vi "writeIMU.vi"(1 "Data":u8 format="%x", 2 "Address":u8 format="%x", 3 "SPI Config In":T1) -> (0 "SPI Config Out":T1)   [LabVIEW 2019]
uses:
  SPI/SPI Config.ctl
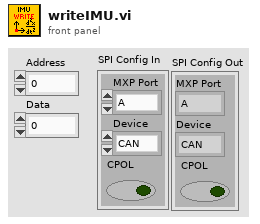
[diagram p1: front panel]
types:
  T1 = typedef "SPI Config.ctl" = cluster{"MXP Port":enum16{"A", "B"}, "Device":enum16{"CAN", "ENC", "IMU1", "IMU2"}, "CPOL":bool}
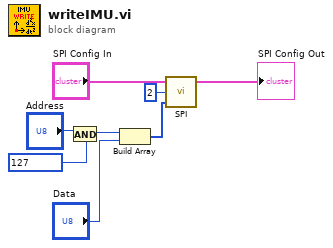
[diagram p0: block diagram]
diagram:
  n1 = And(x="Address", y=u8 127) -> (x .and. y?=w2:u8)
  n2 = Build Array(w2, "Data") -> (w6:u8[])
  n3 = call "SPI.vi"("Data to Write"=w6, "Frames to Write"=u8 2, "SPI Config In"="SPI Config In") -> ("SPI Config Out"=→"SPI Config Out":T1)  [unwired: 2 out]
